vi "solar_voy_def Parse Args (Desc).vi"(11 "Default ITEM":T1) -> (3 "ITEM out":T1)   [LabVIEW 2018]
doc: "This parses a parameter/item description by item modifiers. This is used by Voyager to import the custom LabVIEW data types from the COSMOS definition files. \n\nDescription Arguments\n# lv=LVTYPE, DESCRIPTION - Sets the LabVIEW data type\n\nLVTYPE:\nNative: U8,U16,U32,U64,I8,I16,I32,I64,SGL,DBL,STRING\nCustom: BOOLEAN,PATH,VISA,TAG,TIME,U8_ENUM,U16_ENUM,U32_ENUM\n\n1D Arrays: LVTYPE_1D\n2D Arrays: LVTYPE_2D (Currently not supported)\n\nExamples: \n# lv=<lvtype>, <remaining_description>\n# lv=BOOLEAN, This item is an 8 bit boolean\n# lv=U16_ENUM, This item is an 16 bit enum\n# lv=PATH, This item is a path"
uses:
  solar_voy_def_ctl ITEM TYPE.ctl
  type/solar_type Item Type.ctl
  solar_voy_def_ctl ITEM.ctl
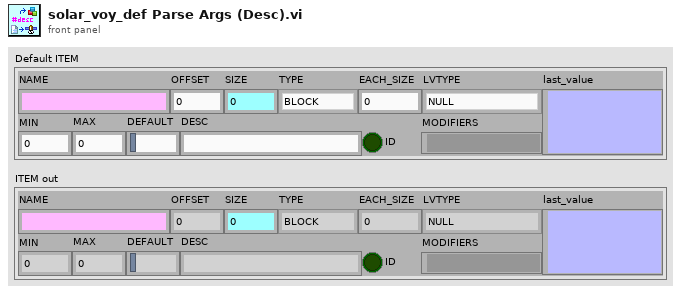
[diagram p1: front panel]
types:
  T1 = typedef "solar_voy_def_ctl ITEM.ctl" = cluster{"NAME":string, "OFFSET":i32, "SIZE":i32, "TYPE":T2, "EACH_SIZE":i32, "LVTYPE":T3, "MIN":dbl, "MAX":dbl, "DEFAULT":string, "DESC":string, "ID":bool, "MODIFIERS":variant, "last_value":variant}
  T2 = typedef "solar_voy_def_ctl ITEM TYPE.ctl" = enum8{"BLOCK", "INT", "UINT", "FLOAT", "STRING"}
  T3 = typedef "solar_type Item Type.ctl" = enum16{"NULL", "UNKNOWN", "CLUSTER", "I8", "I16", "I32", "I64", "U8", "U16", "U32", "U64", "U8_ENUM", "U16_ENUM", "U32_ENUM", "SGL", "DBL", "BOOLEAN", "STRING", "PATH", "VISA", "TAG", "TIME", "I8_1D", "I16_1D", "I32_1D", "I64_1D", "U8_1D", "U16_1D", "U32_1D", "U64_1D", "U8_ENUM_1D", "U16_ENUM_1D", "U32_ENUM_1D", "SGL_1D", "DBL_1D", "BOOLEAN_1D", "STRING_1D", "PATH_1D", "VISA_1D", "TAG_1D", "TIME_1D", "I8_2D", "I16_2D", "I32_2D", "I64_2D", "U8_2D", "U16_2D", "U32_2D", "U64_2D", "U8_ENUM_2D", "U16_ENUM_2D", "U32_ENUM_2D", "SGL_2D", "DBL_2D", "BOOLEAN_2D", "STRING_2D", "PATH_2D", "VISA_2D", "TAG_2D", "TIME_2D"}
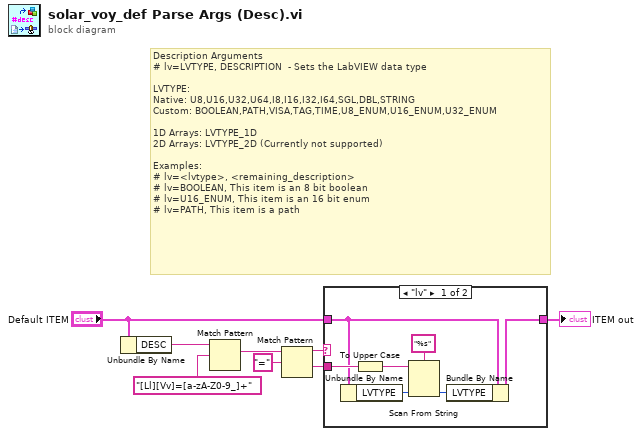
[diagram p0: block diagram]
diagram:
  # "Description Arguments\n# lv=LVTYPE, DESCRIPTION  - Sets the LabVIEW data type\n\nLVTYPE:\nNative: U8,U16,U32,U64,I8,I16,I32,I64,SGL,DBL,STRING\nCustom: BOOLEAN,PATH,VISA,TAG,TIME,U8_ENUM,U16_ENUM,U32_ENUM\n\n1D Arrays: LVTYPE_1D\n2D Arrays: LVTYPE_2D (Currently not supported)\n\nExamples: \n# lv=<lvtype>, <remaining_description>\n# lv=BOOLEAN, This item is an 8 bit boolean\n# lv=U16_ENUM, This item is an 16 bit enum\n# lv=PATH, This item is a path"
  n1 = Unbundle By Name("Default ITEM") -> ("DESC"=w7:string)
  n2 = Match Pattern(string=w7, regular expression="[Ll][Vv]=[a-zA-Z0-9_]+") -> (match substring=w1:string)  [unwired: 1 in, 3 out]
  n3 = Match Pattern(string=w1, regular expression="=") -> (before substring=w3:string, after substring=w2:string)  [unwired: 1 in, 2 out]
  n4 = case shown="\"lv\"" w3 {
    tunnel: [w11 w16] -> w8
    tunnel: "Default ITEM" -> [w14 w16]
    tunnel: w2 -> [w15 _]
    frame "lv" {
      n5 = Unbundle By Name(w14) -> ("LVTYPE"=w13:T3)
      n6 = To Upper Case(1:w15) -> (0:w9:string)
      n7 = Scan From String(format string="%s", input string=w9, default 1=w13) -> (output 1=w10:T3)  [unwired: 2 in, 3 out]
      n8 = Bundle By Name(cluster=w14, "LVTYPE"=w10) -> (w11:T1)
    }
    frame Default {
    }
  }
  "ITEM out" <- w8
